vi "IVCurvePulsed2.vi"(6 "CurrentPositionIndex":i32, 10 "Program":string, 11 "UiDefinition":T3) -> (1 "appended array":dbl[][](array[numeric]), 3 "InfoCluster":T1)   [LabVIEW 2020]
uses:
  UIReferences.ctl
  C:/Users/User/Desktop/Automation/CurrentVersion/LabviewDXFViewer/bin/Release/LabviewDXFViewer.exe
  LabviewDXFViewer/bin/Release/LabviewDXFViewer.exe
  CapacitanceInfos.ctl
  CapacitanceRecord.ctl
  Keithley 2600 Series/Keithley 2600 Series.lvlib
panel:
  out "error out 5":errorcluster
  out "error out 4":errorcluster
  out "error out 3":errorcluster
  out "error out 2":errorcluster
  out "error out":errorcluster
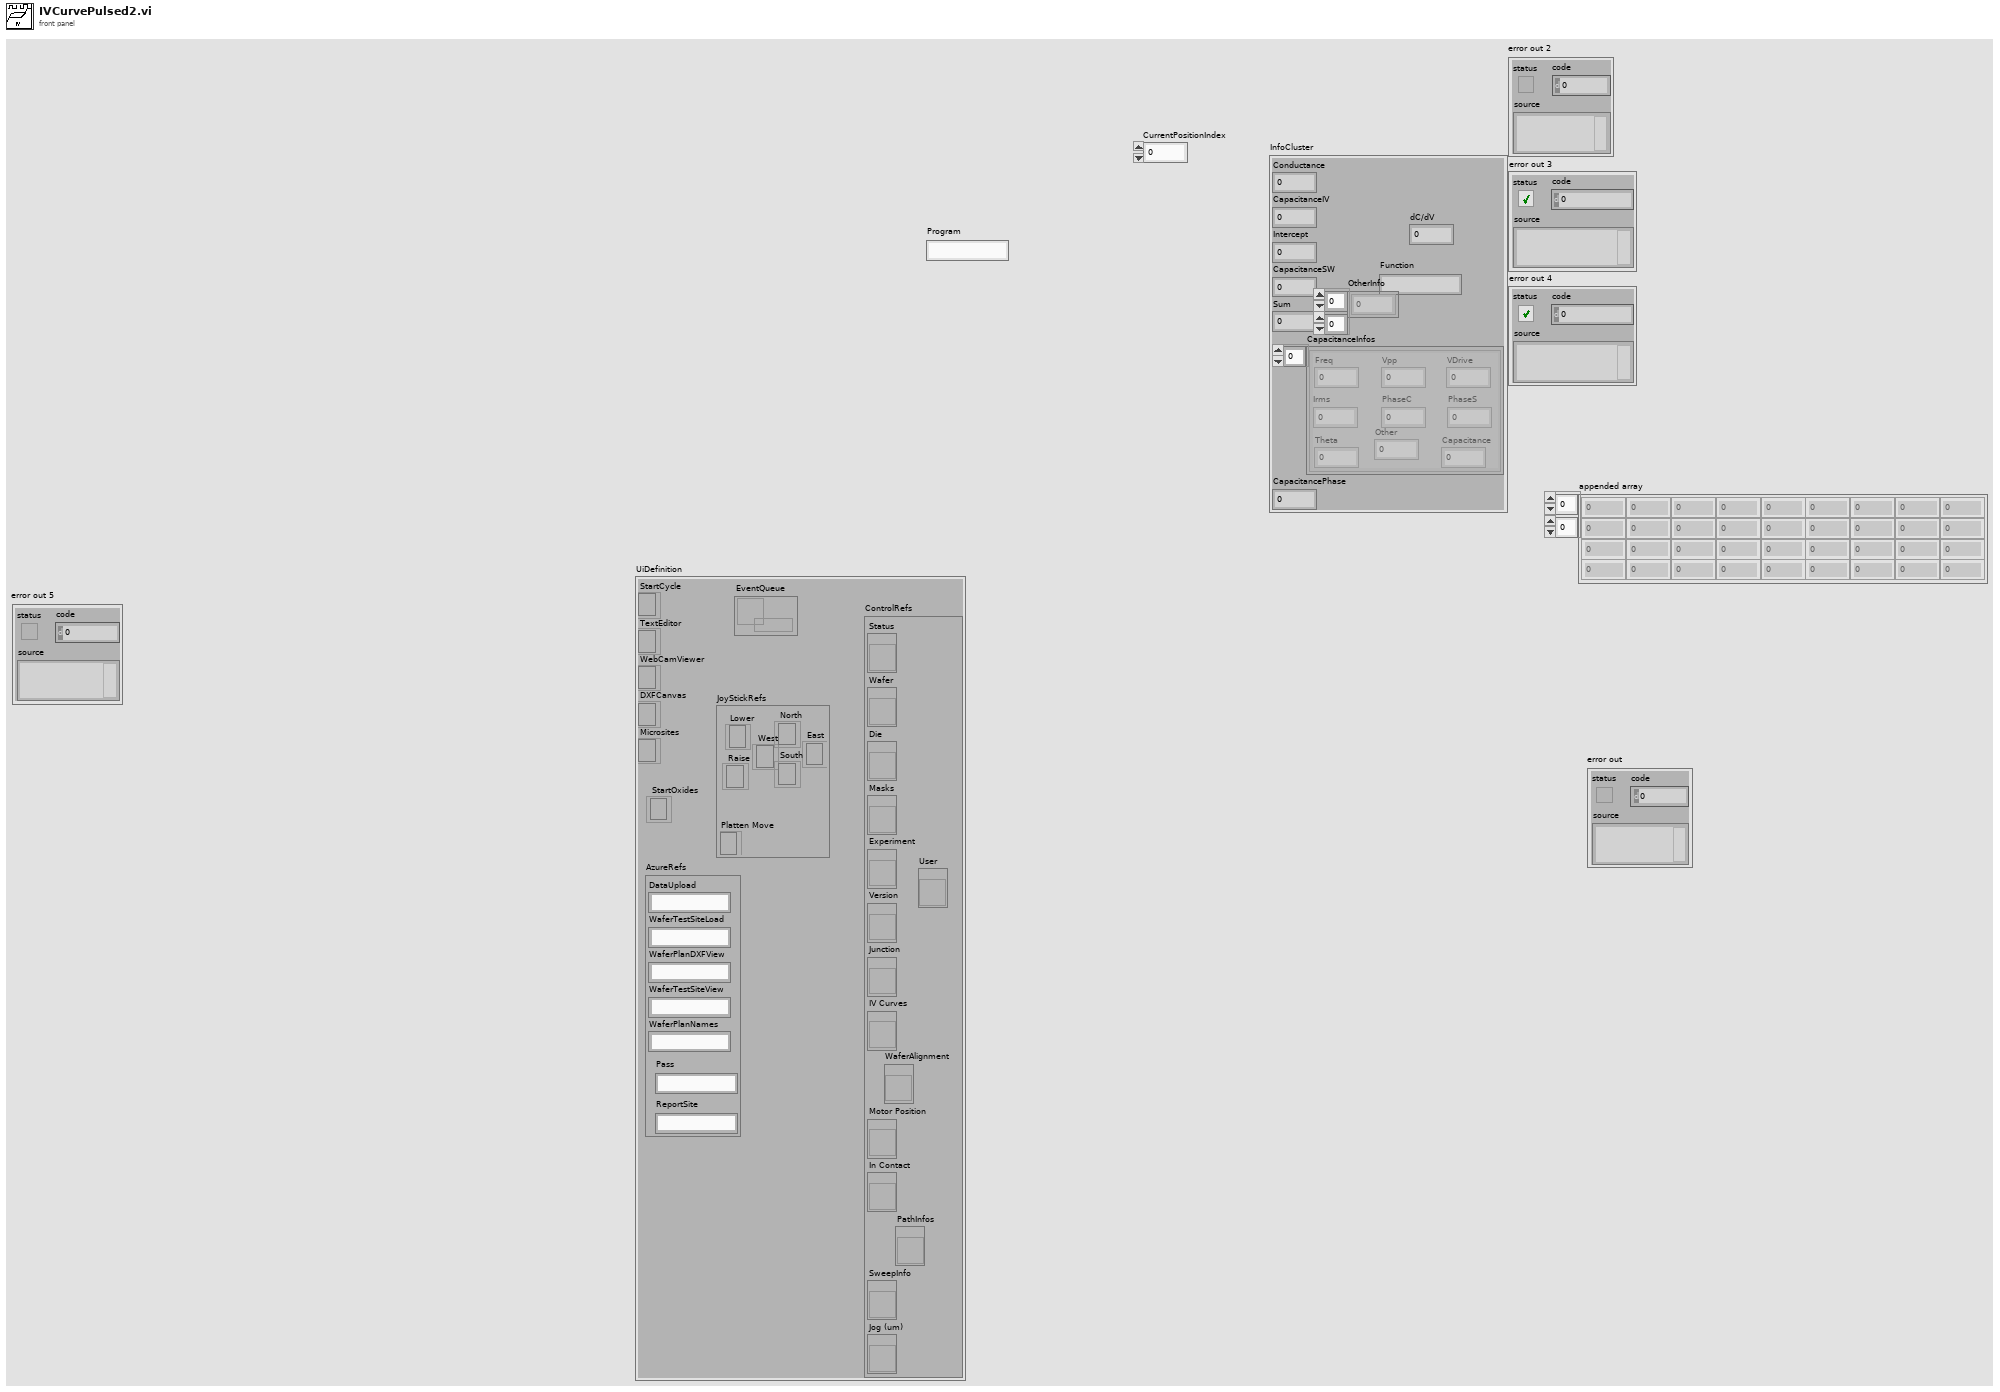
[diagram p1: front panel]
types:
  T1 = typedef "CapacitanceInfos.ctl" = cluster{"Conductance":dbl, "CapacitanceIV":dbl, "Intercept":dbl, "CapacitanceSW":dbl, "Sum":dbl, "CapacitanceInfos":T2[], "CapacitancePhase":dbl, "dC/dV":dbl, "Function":string, "OtherInfo":dbl[][]}
  T2 = typedef "CapacitanceRecord.ctl" = cluster{"Freq":dbl, "Vpp":dbl, "PhaseS":dbl, "Irms":dbl, "PhaseC":dbl, "Theta":dbl, "VDrive":dbl, "Capacitance":dbl, "Other":dbl}
  T3 = typedef "UIReferences.ctl" = cluster{"StartCycle":refnum<k24>, "TextEditor":refnum<k24>, "WebCamViewer":refnum<k24>, "DXFCanvas":refnum<k24>, "Microsites":refnum<k24>, "JoyStickRefs":cluster{"North":refnum<k24>, "Lower":refnum<k24>, "Raise":refnum<k24>, "Platten Move":refnum<k24>, "West":refnum<k24>, "East":refnum<k24>, "South":refnum<k24>}, "AzureRefs":cluster{"DataUpload":string, "WaferTestSiteLoad":string, "WaferPlanDXFView":string, "WaferTestSiteView":string, "WaferPlanNames":string, "Pass":string, "ReportSite":string}, "ControlRefs":cluster{"Status":refnum<vi>, "Wafer":refnum<vi>, "Die":refnum<vi>, "Masks":refnum<vi>, "Experiment":refnum<vi>, "Version":refnum<vi>, "Junction":refnum<vi>, "IV Curves":refnum<vi>, "Motor Position":refnum<vi>, "In Contact":refnum<vi>, "SweepInfo":refnum<vi>, "Jog (um)":refnum<vi>, "PathInfos":refnum<vi>, "User":refnum<vi>, "WaferAlignment":refnum<vi>}, "EventQueue":refnum<queue>, "StartOxides":refnum<k24>}
  T4 = cluster{"Current Range":dbl, "Source Measure Unit Channel (0: Channel A)":i32, "Waveform":waveform(dbl), "VISA resource name":refnum<visa-resource-name>, "CodeText":string}
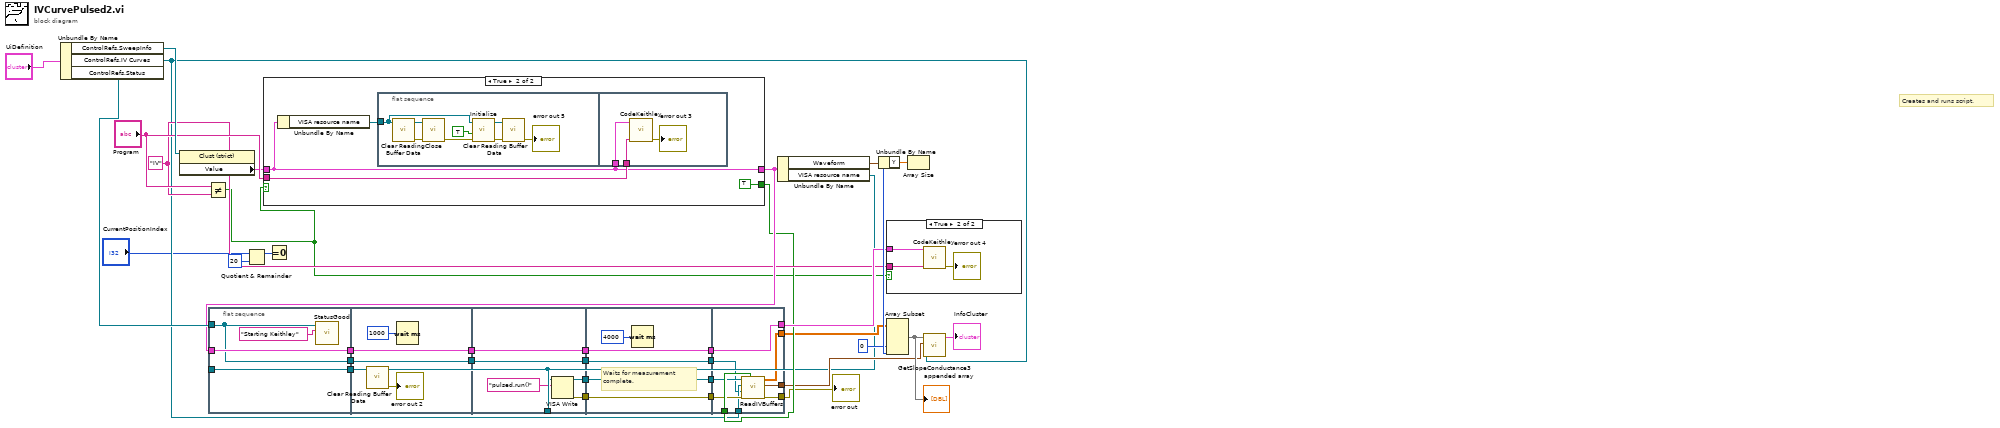
[diagram p0: block diagram]
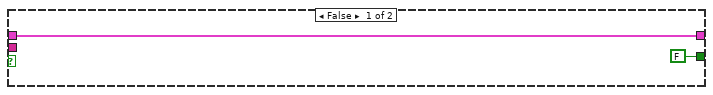
[diagram p3: hidden frame]
diagram:
  w19 = "IV" ("y")
  # "Creates and runs script."
  n1 = Unbundle By Name("UiDefinition") -> ("ControlRefs.SweepInfo"=w35:refnum<vi>, "ControlRefs.IV Curves"=w10:refnum<vi>, "ControlRefs.Status"=w28:refnum<vi>)
  n2 = property class="Clust (strict)"(reference=w35) -> ("Value"=w25:T4)  [unwired: 1 in, 2 out]
  n3 = Not Equal?(x="Program", y=w19) -> (x != y?=w1:bool)
  n4 = flat-sequence {
    tunnel: w9 -> [w41]
    tunnel: [w41] -> w29
    tunnel: w28 -> [w38]
    tunnel: [w39] -> w24
    tunnel: w23 -> [w39]
    tunnel: [w38] -> w5
    tunnel: w29 -> [w45]
    tunnel: w24 -> [w43]
    tunnel: [w43] -> w21
    tunnel: w5 -> [w42]
    tunnel: [w42] -> w4
    tunnel: [w50] -> w37
    tunnel: w9 -> [w51]
    tunnel: [w49] -> w22
    tunnel: w21 -> [w49]
    tunnel: [w48] -> w11
    tunnel: w4 -> [w47]
    tunnel: [w47] -> w3
    tunnel: w37 -> [w57]
    tunnel: w22 -> [w55]
    tunnel: [w57] -> w18
    tunnel: [w55] -> w17
    tunnel: [w54] -> w12
    tunnel: w11 -> [w54]
    tunnel: w3 -> [w53]
    tunnel: [w53] -> w2
    tunnel: [w66] -> w20
    tunnel: w18 -> [w64]
    tunnel: w17 -> [w66]
    tunnel: w16 -> [w65]
    tunnel: w10 -> [w59]
    tunnel: [w63] -> w15
    tunnel: [w62] -> w14
    tunnel: [w61] -> w13
    tunnel: w12 -> [w60]
    tunnel: w2 -> [w58]
    frame #0 {
      n5 = call "StatusGood.vi"("Text.Text"="Starting Keithley", "String in"=w38) -> ()  [unwired: 10 in]
    }
    frame #1 {
      n6 = call "Clear Reading Buffer Data.vi"("VISA resource name"=w45) -> ("error out"=→"error out 2":errorcluster)  [unwired: 9 in, 1 out]
      n7 = Wait (ms)(milliseconds to wait=u32 1000) -> ()  [unwired: 1 out]
    }
    frame #2 {
      n8 = VISA Write(VISA resource name=w51, write buffer="pulsed.run()" ("format string")) -> (VISA resource name out=w50:refnum<visa-resource-name>, error out=w48:errorcluster)  [unwired: 1 in, 1 out]
    }
    frame #3 {
      # "Waits for measurement complete."
      n9 = Wait (ms)(milliseconds to wait=4000) -> ()  [unwired: 1 out]
    }
    frame #4 {
      n10 = call "ReadIVBuffers.vi"("GetCapacitors"=w65, "error in (no error)"=w60, "Status"=w58, "XYGraph Refnum"=w59, "VISA Refnum in"=w64) -> ("error out"=w63:errorcluster, "CapacitanceInfos"=w62:T2[], "Array"=w61:dbl[][])  [unwired: 4 in]
    }
  }
  n11 = Quotient & Remainder(x="CurrentPositionIndex", y=20) -> (x-y*floor(x/y)=w6:i32)  [unwired: 1 out]
  n12 = case shown="True" w1 {
    tunnel: [FALSE TRUE] -> w16
    tunnel: "Program" -> [_ w71]
    tunnel: w25 -> [w67 w70]
    tunnel: [w67 w70] -> w23
    frame False {
    }
    frame True {
      n13 = Unbundle By Name(w70) -> ("VISA resource name"=w69:refnum<visa-resource-name>)
      n14 = flat-sequence {
        tunnel: w69 -> [w73]
        tunnel: w71 -> [w82]
        tunnel: w70 -> [w81]
        frame #0 {
          n15 = call "Clear Reading Buffer Data.vi"("VISA resource name"=w73) -> ("error out"=w80:errorcluster, "VISA resource name out"=w79:refnum<visa-resource-name>)  [unwired: 9 in]
          n16 = call "Close.vi"("error in (no error)"=w80, "VISA resource name"=w79) -> ("error out"=w76:errorcluster)  [unwired: 9 in]
          n17 = call "Initialize.vi"("error in (no error)"=w76, "Reset (True)"=TRUE, "VISA resource name"=w73) -> ("error out"=w77:errorcluster, "VISA resource name out"=w78:refnum<visa-resource-name>)  [unwired: 7 in]
          n18 = call "Clear Reading Buffer Data.vi"("error in (no error)"=w77, "VISA resource name"=w78) -> ("error out"=→"error out 5":errorcluster)  [unwired: 8 in, 1 out]
        }
        frame #1 {
          n19 = call "CodeKeithley.vi"("Program"=w82, "SweepInfo"=w81) -> ("error out"=→"error out 3":errorcluster)  [unwired: 9 in]
        }
      }
    }
  }
  n20 = Equal To 0?(x=w6) -> ()  [unwired: 1 out]
  n21 = Unbundle By Name(w23) -> ("Waveform"=w34:waveform(dbl), "VISA resource name"=w9:refnum<visa-resource-name>)
  n22 = Unbundle By Name(w34) -> ("Y"=w33:dbl[])
  n23 = case shown="True" w1 {
    tunnel: w19 -> [_ w86]
    tunnel: w20 -> [_ w85]
    frame False {
    }
    frame True {
      n24 = call "CodeKeithley.vi"("Program"=w86, "SweepInfo"=w85) -> ("error out"=→"error out 4":errorcluster)  [unwired: 9 in]
    }
  }
  n25 = Array Size(array=w33) -> (size(s)=w32:i32)
  n26 = Array Subset(array=w13, index (col)=0 ("index"), length (col)=w32) -> (w30:dbl[][])  [unwired: 2 in]
  "appended array" <- w30
  n27 = call "GetSlopeConductance3.vi"("XYGraph Refnum"=w10, "CapacitanceRecords"=w14, "Array in"=w30) -> ("InfoCluster"=→"InfoCluster":T1)  [unwired: 7 in, 1 out]
  "error out" <- w15
